vi "Pack for gRPC.vi"(8 "error in (no error)":errorcluster, 9 "Configuration / Resuls (Config)":enum16{"Configuration", "Results"}(ring), 10 "Data Value":variant, 11 "Measurement Customizations in":refnum<class "MeasurementPlugin.lvclass">) -> (0 "error out":errorcluster, 2 "Any":T1, 3 "Measurement Customizations out":refnum<class "MeasurementPlugin.lvclass">)   [LabVIEW 2022 SP3, in "Single Tone No Gen_Class D Amplifier.lvlib" / "MeasurementPlugin.lvclass"]
uses:
  MeasurementPlugin.lvclass
  MeasurementPlugin.lvclass/MeasurementPlugin.ctl
  Measurement Configuration.ctl
  Single Tone No Gen_Class D Amplifier.lvlib
  Measurement Results.ctl
  a6012965-5700-4384-8228-972e71b6560c.vi
  2eca732d-dbaa-43bf-a7dd-ede2da65bc1b.vi
  shared/controls/highpass filter.ctl
  shared/controls/lowpass filter.ctl
  shared/controls/weighting filter.ctl
  shared/controls/units - ratio.ctl
  shared/controls/audio controls.lvlib
  shared/controls/units - snr.ctl
  <vilib>/Plug-In SDKs/Measurements/Measurement Plugin Service/Measurement Plugin Service.lvclass
  C:/Program Files/National Instruments/LabVIEW 2022/vi.lib/Plug-In SDKs/Measurements/Measurement Plugin Service/Measurement Plugin Service.lvclass
  C:/dev/class-d-amplifier/source/single tone no gen/Single Tone No Gen_Class D Amplifier/Advanced/MeasurementPlugin.lvclass
  <vilib>/gRPC/LabVIEW gRPC Library/Shared/Any.ctl
  <vilib>/gRPC/LabVIEW gRPC Library/grpc-lvsupport-release.lvlib
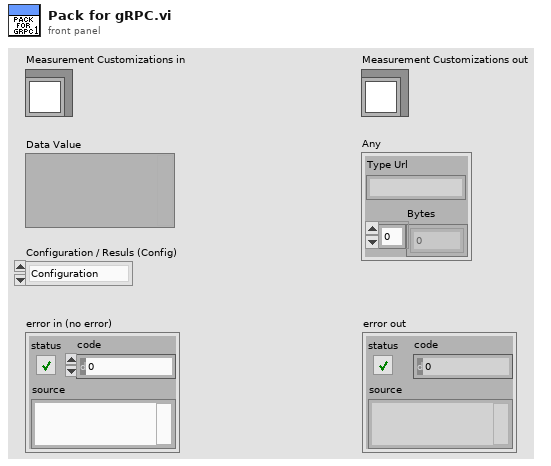
[diagram p1: front panel]
types:
  T1 = typedef "grpc-lvsupport-release.lvlib/Any.ctl" = cluster{"Type Url":string, "Bytes":u8[]}
  T2 = typedef "grpc-lvsupport-release.lvlib/grpcId.ctl" = u64
  T3 = typedef "Single Tone No Gen_Class D Amplifier.lvlib/Measurement Configuration.ctl" = cluster{"input configuration file":string, "digital channel list":string, "analog input channel":string, "min measurement cycles":u32, "min measurement time (s)":dbl, "min settling cycles":u32, "min settling time (s)":dbl, "band start":dbl, "band stop":dbl, "weighting filter":T4, "lowpass filter":T5, "highpass filter":T6, "SNR units":T7, "THD+N units":T8, "THD units":T8, "gain units":T8, "expected amplitude (Vpk)":dbl, "expected signal frequency":dbl, "amplitude reference (Vpk-pk)":dbl, "load impedance":dbl}
  T4 = typedef "weighting filter.ctl" = enum32{"Linear", "A-weighting", "B-weighting", "C-weighting"}
  T5 = typedef "lowpass filter.ctl" = enum32{"No filter", "AES17 20kHz", "AES17 40kHz"}
  T6 = typedef "highpass filter.ctl" = enum32{"DC", "AC"}
  T7 = typedef "audio controls.lvlib/units - snr.ctl" = enum32{"dB", "x/y"}
  T8 = typedef "audio controls.lvlib/units - ratio.ctl" = enum32{"dB", "%", "x/y"}
  T9 = typedef "Single Tone No Gen_Class D Amplifier.lvlib/Measurement Results.ctl" = cluster{"channel names":string[], "frequency (Hz)":dbl[], "amplitude (Vrms)":dbl[], "amplitude (dBFS)":dbl[], "phase (deg)":dbl[], "SNR":dbl[], "THD+N":dbl[], "THD":dbl[], "dynamic range (dB)":dbl[], "gain":dbl[], "SFDR (dBc)":dbl[], "output power (W)":dbl[], "wfm - t0":dbl, "wfm - dt":dbl, "wfm - data":dbl[], "fft - f0":dbl, "fft - df":dbl, "fft - data":dbl[]}
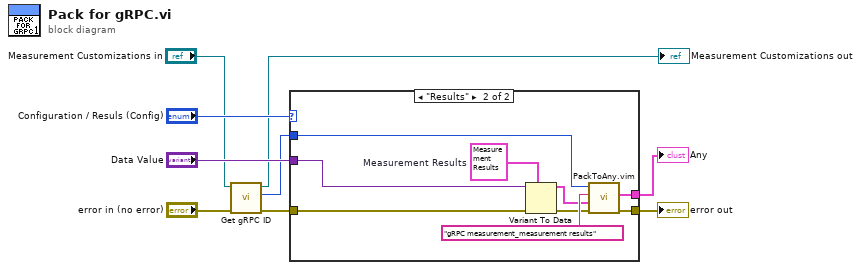
[diagram p0: block diagram]
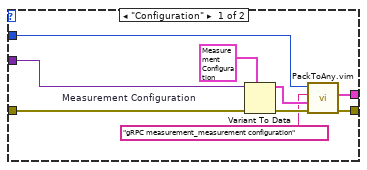
[diagram p2: hidden frame]
diagram:
  n1 = call <vilib>:"Get gRPC ID.vi"("error in"="error in (no error)", "measurement plugin service in"="Measurement Customizations in") -> ("error out"=w4:errorcluster, "gRPC ID"=w1:T2, "measurement plugin service out"=→"Measurement Customizations out":refnum<class "MeasurementPlugin.lvclass">)  [unwired: 7 in]
  n2 = case shown="\"Results\"" "Configuration / Resuls (Config)" {
    tunnel: w4 -> [w18 w27]
    tunnel: "Data Value" -> [w17 w26]
    tunnel: w1 -> [w14 w22]
    tunnel: [w16 w24] -> w8
    tunnel: [w15 w23] -> w7
    frame "Configuration" {
      w11 = T3 {"input configuration file"="", "digital channel list"="7821\\PCMo 8", "analog input channel"="", "min measurement cycles"=1000, "min measurement time (s)"=5.0, "min settling cycles"=0, "min settling time (s)"=0.0, "band start"=20.0, "band stop"=20000.0, "weighting filter"=enum."Linear", "lowpass filter"=enum."No filter", "highpass filter"=enum."DC", "SNR units"=enum."dB", "THD+N units"=enum."dB", "THD units"=enum."dB", "gain units"=enum."dB", "expected amplitude (Vpk)"=48000.0, "expected signal frequency"=1000.0, "amplitude reference (Vpk-pk)"=2.0, "load impedance"=4.0}  # Measurement Configuration
      n3 = Variant To Data(error in=w18, type=w11, Variant=w17) -> (data=w13:T3, error out=w12:errorcluster)
      n4 = call "PackToAny.vim"("error in"=w12, "Data To Pack"=w13, "Message Type"="gRPC measurement_measurement configuration", "gRPCid in"=w14) -> ("error out"=w16:errorcluster, "Any"=w15:T1)  [unwired: 5 in, 1 out]
    }
    frame "Results" {
      w25 = T9 {"channel names"=[], "frequency (Hz)"=[], "amplitude (Vrms)"=[], "amplitude (dBFS)"=[], "phase (deg)"=[], "SNR"=[], "THD+N"=[], "THD"=[], "dynamic range (dB)"=[], "gain"=[], "SFDR (dBc)"=[], "output power (W)"=[], "wfm - t0"=0.0, "wfm - dt"=0.0, "wfm - data"=[], "fft - f0"=0.0, "fft - df"=0.0, "fft - data"=[]}  # Measurement Results
      n5 = Variant To Data(error in=w27, type=w25, Variant=w26) -> (data=w20:T9, error out=w19:errorcluster)
      n6 = call "PackToAny.vim"("error in"=w19, "Data To Pack"=w20, "Message Type"="gRPC measurement_measurement results", "gRPCid in"=w22) -> ("error out"=w24:errorcluster, "Any"=w23:T1)  [unwired: 5 in, 1 out]
    }
  }
  "error out" <- w8
  "Any" <- w7
